vi "Get Groups.vi"(8 "error in (no error)":errorcluster, 11 "Plugin Ref in":T1 format="%.0x") -> (0 "error out":errorcluster, 2 "Group refs":T1[](array[typedef]) format="%.0x", 3 "Plugin Ref out":T1 format="%.0x")   [LabVIEW 2021, in "DSF Shared.lvlib"]
uses:
  DSF Shared.lvlib
  <vilib>/NI VeriStand/Custom Device API/Custom Device Item Ref.ctl
  Group Page GUID.vi
  <vilib>/NI VeriStand/Custom Device API/Custom Device API.lvlib
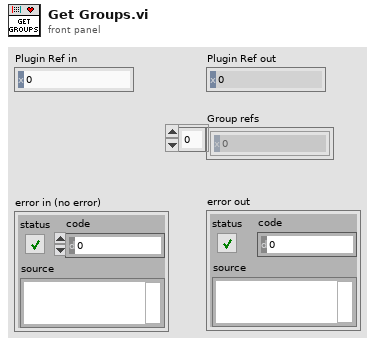
[diagram p1: front panel]
types:
  T1 = typedef "Custom Device API.lvlib/Custom Device Item Ref.ctl" = u64
  T2 = typedef "Custom Device API.lvlib/Custom Device Item Info.ctl" = cluster{"Name":string, "Is Channel":bool, "GUID":string, "Is Waveform":bool}
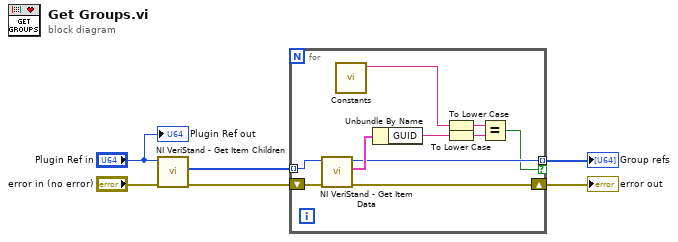
[diagram p0: block diagram]
diagram:
  n1 = call <vilib>:"NI VeriStand - Get Item Children.vi"("error in (no error)"="error in (no error)", "Item Ref in"="Plugin Ref in") -> ("error out"=w5:errorcluster, "Child Refs"=w3:T1[])  [unwired: 6 in, 2 out]
  n2 = for {
    shift-right: [w15] -> w2
    shift-left: w5 -> [w16]
    tunnel: w3 -> [w13] mode=indexing
    tunnel: [w11] -> w1 mode=indexing if=w10
    n3 = call <vilib>:"NI VeriStand - Get Item Data.vi"("error in (no error)"=w16, "Item Ref in"=w13) -> ("error out"=w15:errorcluster, "Item Info"=w14:T2, "Item Ref out"=w11:T1)  [unwired: 6 in, 1 out]
    n4 = call-poly "Constants.vi"() -> ("Group GUID"=w9:string)  [unwired: 11 in]
    n5 = Unbundle By Name(w14) -> ("GUID"=w12:string)
    n6 = To Lower Case(string=w9) -> (all lower case string=w8:string)
    n7 = To Lower Case(string=w12) -> (all lower case string=w7:string)
    n8 = Equal?(x=w8, y=w7) -> (x = y?=w10:bool)
  }
  "error out" <- w2
  "Group refs" <- w1
  "Plugin Ref out" <- "Plugin Ref in"
